vi "Get Data Acquisition Done Status.vi"(4 "error in (no error)":errorcluster, 7 "VISA resource name":refnum<visa-resource-name>) -> (0 "error out":errorcluster, 2 "Data acquisition status":bool, 3 "VISA resource name out":refnum<visa-resource-name>)   [LabVIEW 2015, in "Newport ESP301.lvlib"]
doc: "Returns the status of a data acquisition request."
uses:
  Newport ESP301.lvlib
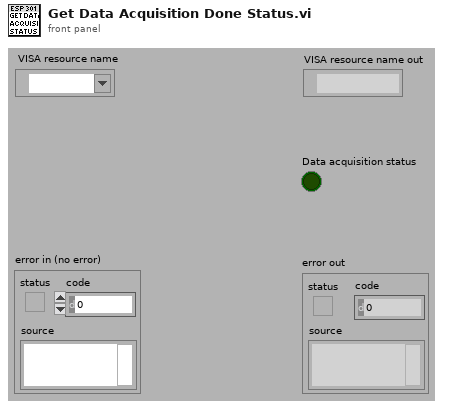
[diagram p1: front panel]
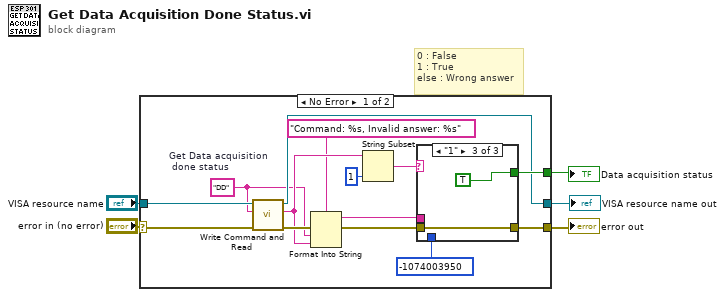
[diagram p0: block diagram]
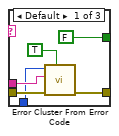
[diagram p2: hidden frame]
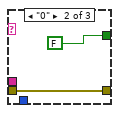
[diagram p3: hidden frame]
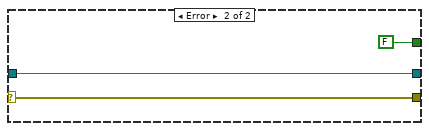
[diagram p4: hidden frame]
diagram:
  # "0 : False\n1 : True\nelse : Wrong answer"
  n1 = case shown="No Error" "error in (no error)" {
    selector: "error in (no error)" -> [w18 w32]
    tunnel: [w12 w32] -> w5
    tunnel: "VISA resource name" -> [w19 w31]
    tunnel: [w13 w31] -> w4
    tunnel: [w14 FALSE ("Motion Done")] -> w1
    frame No Error {
      w6 = "DD"  # Get Data acquisition  done status
      n2 = call "Write Command and Read.vi"("error in (no error)"=w18, "Command"=w6, "VISA resource name"=w19) -> ("error out"=w10:errorcluster, "Returned string"=w8:string, "VISA resource name out"=w13:refnum<visa-resource-name>)  [unwired: 2 in, 2 out]
      n3 = Format Into String(format string="Command: %s, Invalid answer: %s" ("error message (\"\")"), error in=w10, w6, w8) -> (resulting string=w15:string, error out=w9:errorcluster)  [unwired: 1 in]
      n4 = String Subset(string=w8, length (rest)=1 ("longueur (reste)")) -> (substring=w16:string)  [unwired: 1 out]
      n5 = case shown="\"1\"" w16 {
        tunnel: [w24 w26 w28] -> w12
        tunnel: [FALSE ("Motion Done") FALSE ("Motion Done") TRUE ("Motion Done")] -> w14
        tunnel: w15 -> [w22 _ _]
        tunnel: w9 -> [w21 w26 w28]
        tunnel: -1074003950 ("error code (0)") -> [w20 _ _]
        frame Default {
          n6 = call <vilib>:"Error Cluster From Error Code.vi"("show call chain? (False)"=TRUE, "error in (no error)"=w21, "error message (\"\")"=w22, "error code (0)"=w20) -> ("error out"=w24:errorcluster)  [unwired: 5 out]
        }
        frame "0" {
        }
        frame "1" {
        }
      }
    }
    frame Error {
    }
  }
  "error out" <- w5
  "VISA resource name out" <- w4
  "Data acquisition status" <- w1
